vi "UpdateWaveformWidth.vi"(8 "error in (no error)":errorcluster, 9 "Source bitwidth":u32, 10 "Capture bitwidth":u32, 11 "IVI Refnum in":refnum<k15>) -> (0 "error out":errorcluster, 3 "IVI Refnum out":refnum<k15>)   [LabVIEW 2023]
uses:
  <instrlib>/niDigital/niDigital.llb/niDigital Data Mapping.ctl
  <instrlib>/niDigital/niDigital.llb/niDigital Bit Order.ctl
  <instrlib>/niDigital/niDigital.llb/niDigital Create Capture Waveform (Serial).vi
  <instrlib>/niDigital/niDigital.llb/niDigital Create Source Waveform (Serial).vi
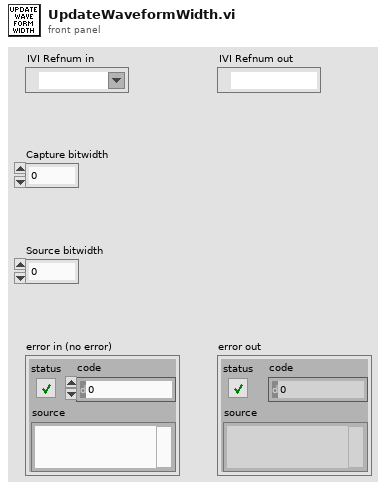
[diagram p1: front panel]
types:
  T1 = typedef "niDigital Bit Order.ctl" = i32
  T2 = typedef "niDigital Data Mapping.ctl" = i32
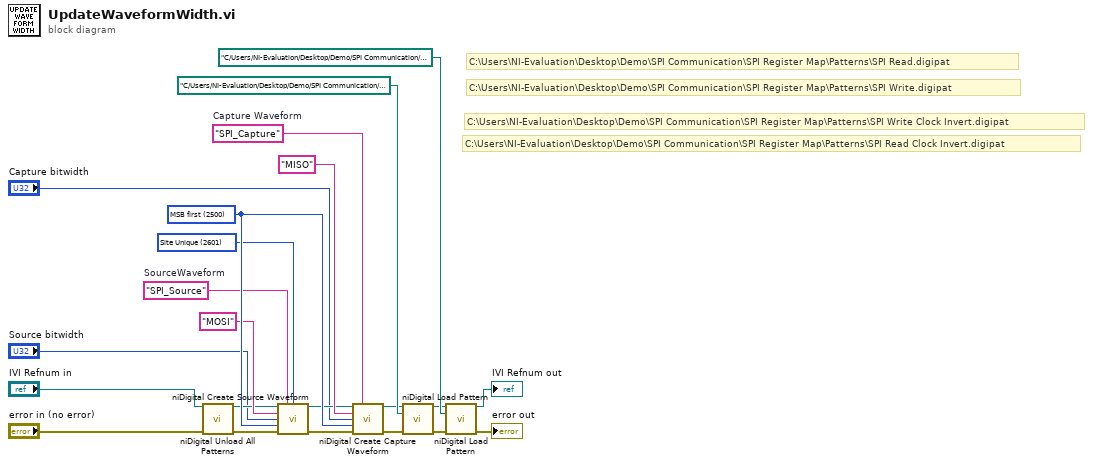
[diagram p0: block diagram]
diagram:
  w16 = T1 2500 items=["MSB first"=2500, "LSB first"=2501] ("bit order")
  w13 = T2 2601 items=["Broadcast"=2600, "Site Unique"=2601] ("data mapping")
  w12 = "SPI_Source"  # SourceWaveform
  w11 = "SPI_Capture"  # Capture Waveform
  # "C:\\Users\\NI-Evaluation\\Desktop\\Demo\\SPI Communication\\SPI Register Map\\Patterns\\SPI Write Clock Invert.digipat"
  # "C:\\Users\\NI-Evaluation\\Desktop\\Demo\\SPI Communication\\SPI Register Map\\Patterns\\SPI Write.digipat"
  # "C:\\Users\\NI-Evaluation\\Desktop\\Demo\\SPI Communication\\SPI Register Map\\Patterns\\SPI Read Clock Invert.digipat"
  # "C:\\Users\\NI-Evaluation\\Desktop\\Demo\\SPI Communication\\SPI Register Map\\Patterns\\SPI Read.digipat"
  n1 = call <instrlib>:"niDigital Unload All Patterns.vi"("instrument handle"="IVI Refnum in", "error in"="error in (no error)") -> ("instrument handle out"=w5:refnum<k15>, "error out"=w6:errorcluster)  [unwired: 12 in]
  n2 = call-poly <instrlib>:"niDigital Create Source Waveform.vi"("instrument handle"=w5, "waveform name"=w12, "data mapping"=w13, "pin list"="MOSI", "sample width"="Source bitwidth", "bit order"=w16, "error in"=w6) -> ("instrument handle out"=w7:refnum<k15>, "error out"=w8:errorcluster)  [unwired: 7 in]
  n3 = call-poly <instrlib>:"niDigital Create Capture Waveform.vi"("instrument handle"=w7, "waveform name"=w11, "pin list"="MISO", "sample width"="Capture bitwidth", "bit order"=w16, "error in"=w8) -> ("instrument handle out"=w3:refnum<k15>, "error out"=w4:errorcluster)  [unwired: 8 in]
  n4 = call <instrlib>:"niDigital Load Pattern.vi"("instrument handle"=w3, "pattern file"=path "C:/Users/NI-Evaluation/Desktop/Demo/SPI Communication/SPI Register Map/Patterns/SPI Write Clock Invert.digipat", "error in"=w4) -> ("instrument handle out"=w17:refnum<k15>, "error out"=w18:errorcluster)  [unwired: 11 in]
  n5 = call <instrlib>:"niDigital Load Pattern.vi"("instrument handle"=w17, "pattern file"=path "C:/Users/NI-Evaluation/Desktop/Demo/SPI Communication/SPI Register Map/Patterns/SPI Read Clock Invert.digipat", "error in"=w18) -> ("instrument handle out"=→"IVI Refnum out":refnum<k15>, "error out"=→"error out":errorcluster)  [unwired: 11 in]
